vi "Get Device Info.vi"(8 "error in (no error)":errorcluster, 11 "RIO Device":T1) -> (0 "error out":errorcluster, 1 "SI Channels":string[](array[string]), 2 "SI Count":i32, 3 "Module Name":string)   [LabVIEW 2025, in "I2C Bus Monitor UI.lvlib"]
uses:
  I2C Bus Monitor UI.lvlib
  <vilib>/userDefined/Silver/nirio_resource_slv.ctl
  <vilib>/nisyscfg/Close (Filter).vi
  <vilib>/nisyscfg/Close (System).vi
  <vilib>/nisyscfg/Close (Hardware).vi
  Error Global.vi
  <vilib>/nisyscfg/nisyscfg.lvlib
  <resource>/objmgr/niflexrioatomicsae.rc
  <resource>/objmgr/nicriosae.rc
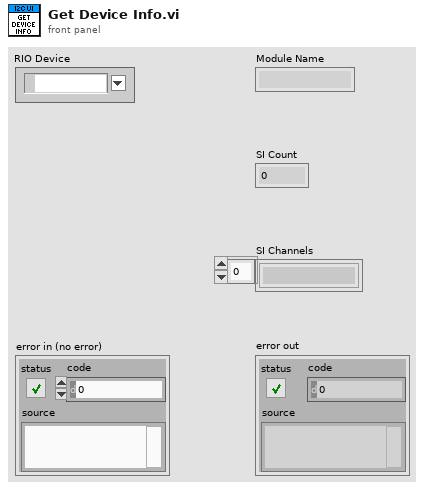
[diagram p1: front panel]
types:
  T1 = typedef "nirio_resource_slv.ctl" = tag
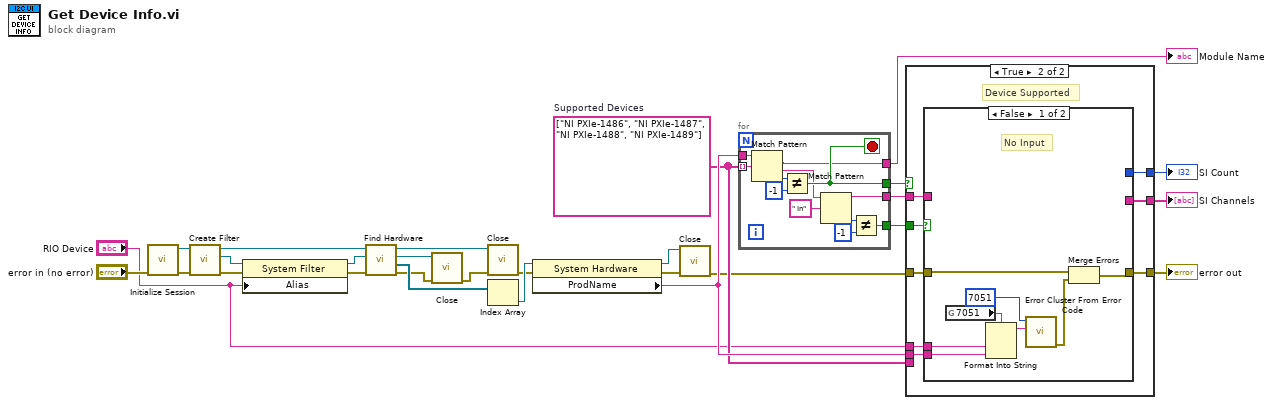
[diagram p0: block diagram]
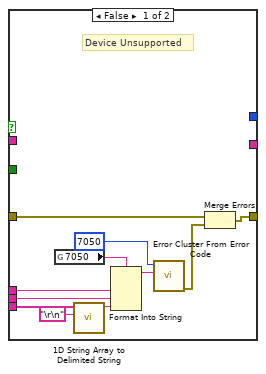
[diagram p2: hidden frame]
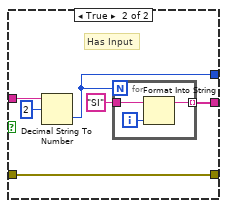
[diagram p3: hidden frame]
diagram:
  w9 = string[] ["NI PXIe-1486", "NI PXIe-1487", "NI PXIe-1488", "NI PXIe-1489"]  # Supported Devices
  n1 = call <vilib>:"Initialize Session.vi"("error in (no error)"="error in (no error)") -> ("error out"=w20:errorcluster, "Session out"=w18:refnum<k21>)  [unwired: 9 in]
  n2 = call <vilib>:"Create Filter.vi"("error in (no error)"=w20, "Session in"=w18) -> ("error out"=w15:errorcluster, "Filter out"=w16:refnum<k20>, "Session out"=w19:refnum<k21>)  [unwired: 7 in]
  n3 = property class="System Filter"(reference=w16, error in=w15, "Alias"="RIO Device") -> (reference out=w17:refnum<k20>, error out=w21:errorcluster)
  n4 = call <vilib>:"Find Hardware.vi"("error in (no error)"=w21, "Filter in"=w17, "Session in"=w19) -> ("error out"=w5:errorcluster, "Resources out"=w14:refnum<k20>[], "Filter out"=w4:refnum<k20>, "Session out"=w13:refnum<k21>)  [unwired: 5 in]
  n5 = call-poly <vilib>:"Close.vi"("error in (no error)"=w5, "Filter in"=w4) -> ("error out"=w3:errorcluster)  [unwired: 9 in]
  n6 = call-poly <vilib>:"Close.vi"("error in (no error)"=w3, "Session in"=w13) -> ("error out"=w12:errorcluster)  [unwired: 9 in]
  n7 = Index Array(array=w14) -> (element=w22:refnum<k20>)  [unwired: 1 in]
  n8 = property class="System Hardware"(reference=w22, error in=w12) -> (reference out=w8:refnum<k20>, error out=w7:errorcluster, "ProdName"=w10:string)
  n9 = call-poly <vilib>:"Close.vi"("error in (no error)"=w7, "Resource in"=w8) -> ("error out"=w6:errorcluster)  [unwired: 9 in]
  n10 = for {
    tunnel: w9 -> [w34] mode=indexing
    tunnel: w10 -> [w40]
    tunnel: [w37] -> w11
    tunnel: [w33] -> w26
    tunnel: [w31] -> w23
    tunnel: [w30] -> w25
    stop <- w37 stop-if-true
    n11 = Match Pattern(string=w40, regular expression=w34) -> (match substring=w33:string, after substring=w29:string, offset past match=w39:i32)  [unwired: 1 in, 1 out]
    n12 = Not Equal?(x=w39, y=-1) -> (x != y?=w37:bool)
    n13 = Match Pattern(string=w29, regular expression=" In") -> (before substring=w31:string, offset past match=w35:i32)  [unwired: 1 in, 2 out]
    n14 = Not Equal?(x=w35, y=-1) -> (x != y?=w30:bool)
  }
  "Module Name" <- w26
  n15 = case shown="True" w11 {
    tunnel: [_ w59] -> w27
    tunnel: w25 -> [_ w58]
    tunnel: [_ w57] -> w24
    tunnel: w23 -> [_ w56]
    tunnel: w6 -> [w45 w55]
    tunnel: [w44 w54] -> w1
    tunnel: w10 -> [w42 w53]
    tunnel: w9 -> [w50 _]
    tunnel: "RIO Device" -> [w41 w52]
    frame False {
      # "Device Unsupported"
      n16 = global read "Error Global.vi" "7050"() -> (w51:string)
      n17 = call <vilib>:"1D String Array to Delimited String.vi"("delimiter"="\r\n", "string array"=w50) -> ("delimited string"=w48:string)  [unwired: 9 in]
      n18 = Format Into String(format string=w51, w41, w42, w48) -> (resulting string=w47:string)  [unwired: 2 in, 1 out]
      n19 = call <vilib>:"Error Cluster From Error Code.vi"("error message (\"\")"=w47, "error code (0)"=7050) -> ("error out"=w43:errorcluster)  [unwired: 7 in]
      n20 = Merge Errors(w45, w43) -> (w44:errorcluster)
    }
    frame True {
      # "Device Supported"
      n21 = case shown="False" w58 {
        tunnel: w56 -> [_ w73]
        tunnel: [_ w71] -> w59
        tunnel: [_ w69] -> w57
        tunnel: w55 -> [w63 w68]
        tunnel: [w62 w68] -> w54
        tunnel: w53 -> [w61 _]
        tunnel: w52 -> [w60 _]
        frame False {
          # "No Input"
          n22 = global read "Error Global.vi" "7051"() -> (w67:string)
          n23 = Format Into String(format string=w67, w60, w61) -> (resulting string=w66:string)  [unwired: 2 in, 1 out]
          n24 = call <vilib>:"Error Cluster From Error Code.vi"("error message (\"\")"=w66, "error code (0)"=7051) -> ("error out"=w64:errorcluster)  [unwired: 7 in]
          n25 = Merge Errors(w63, w64) -> (w62:errorcluster)
        }
        frame True {
          # "Has Input"
          n26 = Decimal String To Number(string=w73, offset=2) -> (number=w71:i32)  [unwired: 1 in, 1 out]
          n27 = for {
            N: w71 -> [_]
            tunnel: "SI" -> [w76]
            tunnel: [w74] -> w69 mode=indexing
            i -> [w75]
            n28 = Format Into String(initial string=w76, w75) -> (resulting string=w74:string)  [unwired: 2 in, 1 out]
          }
        }
      }
    }
  }
  "SI Count" <- w27
  "SI Channels" <- w24
  "error out" <- w1
